vi "Global Variable_Waveforms.vi"() -> ()   [LabVIEW 2012]
panel:
  in  "Gate Wavefprm (digital)":digitalwaveform(waveform)
  in  "Pockels Waveform":waveform(dbl)
  in  "XY Waveform":waveform(dbl)[](array[waveform])=[{"t0"=timestamp(0 s since 1904-01-01), "dt"=1e-05, "Y"=array[162020 elements]}, {"t0"=timestamp(0 s since 1904-01-01), "dt"=1e-05, "Y"=array[162020 elements]}]
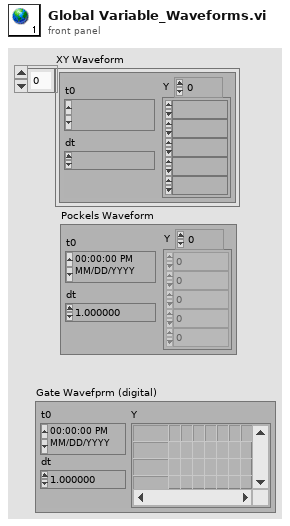
[diagram p1: front panel]
diagram:
